vi "Server - Main.vi"(8 "error in (no error)":errorcluster) -> (0 "error out":errorcluster)   [LabVIEW 2019]
doc: "This VI runs on the server."
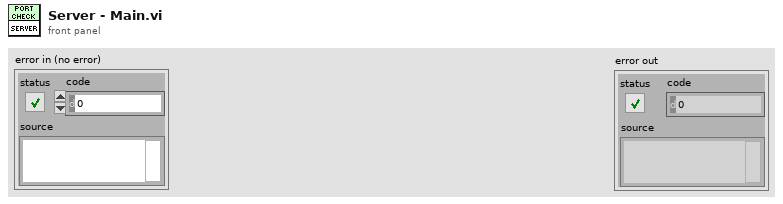
[diagram p1: front panel]
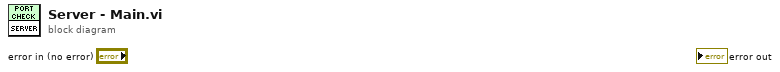
[diagram p0: block diagram]
diagram:
